vi "LoadParameters.vi"(11 "ShiftConfigPath":path) -> (3 "JSON_Text":string)   [LabVIEW 2017]
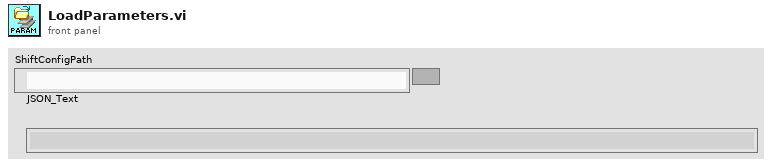
[diagram p1: front panel]
types:
  T1 = enum16{"open", "replace", "create", "open or create", "replace or create", "replace or create with confirmation"}
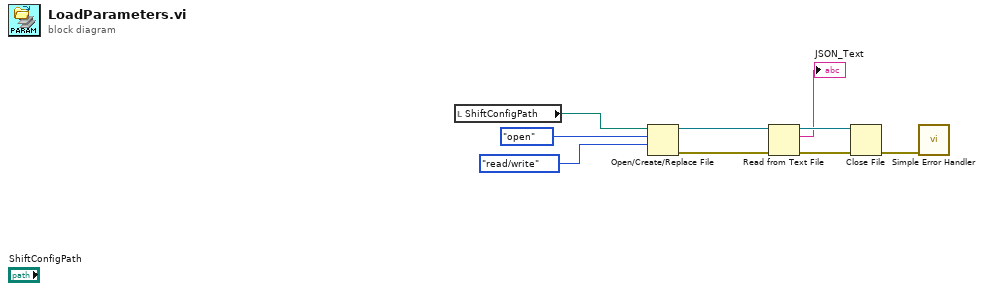
[diagram p0: block diagram]
diagram:
  n1 = local read "ShiftConfigPath"() -> (w2:path)
  n2 = Open/Create/Replace File(file path (use dialog)=w2, operation (0:open)=T1."open", access (0:read/write)=enum16{"read/write", "read-only", "write-only"}."read/write") -> (refnum out=w9:refnum<file>, error out=w8:errorcluster)  [unwired: 3 in, 1 out]
  n3 = Read from Text File(file (use dialog)=w9, error in=w8) -> (refnum out=w6:refnum<file>, text=→"JSON_Text":string, error out=w5:errorcluster)  [unwired: 2 in, 1 out]
  n4 = Close File(refnum=w6, error in=w5) -> (error out=w4:errorcluster)  [unwired: 1 out]
  n5 = call <vilib>:"Simple Error Handler.vi"("error in (no error)"=w4) -> ()  [unwired: 4 in, 5 out]
